vi "Text Description.vi"(11 "SubstututeMessage in":refnum<class "SubstututeMessage.lvclass">) -> (2 "Description":string, 3 "SubstututeMessage out":refnum<class "SubstututeMessage.lvclass">)   [LabVIEW 2011, in "Messenging.lvlib" / "SubstututeMessage.lvclass"]
uses:
  SubstututeMessage.lvclass
  TextVarientMessage/MSG.lvclass
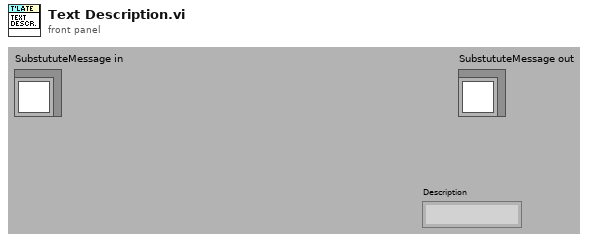
[diagram p1: front panel]
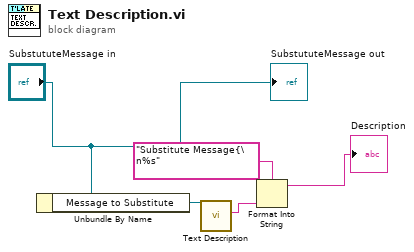
[diagram p0: block diagram]
diagram:
  n1 = Unbundle By Name("SubstututeMessage in") -> ("Message to Substitute"=w5:refnum<class "MSG.lvclass">)
  n2 = call-dynamic "Text Description.vi"("Message"=w5) -> ("Description"=w3:string)  [unwired: 10 out]
  n3 = Format Into String(format string="Substitute Message{\n%s", w3) -> (resulting string=→"Description":string)  [unwired: 2 in, 1 out]
  "SubstututeMessage out" <- "SubstututeMessage in"
